vi "Two Color Calibration.vi"(7 "Calling VI Ref":refnum<vi>) -> ()   [LabVIEW 2016]
uses:
  <vilib>/Utility/miscctls.llb/LVPointTypeDef.ctl
  Hardware Configuration/Hardware Configuration Controls/Device Type.ctl
  Hardware Configuration/Hardware Configuration Controls/Device Function.ctl
  Two Color Cal Type Defs/Two Color Cal Notifier Type.ctl
  Two Color Cal Type Defs/Two Color Cal Actions.ctl
  Tools/TIFF Image Read and Write/ImageJ TIF Type Defs/TIF Write Image Information.ctl
  Device Library/Cameras/Camera Controls/Generic Camera Actions.ctl
  Device Library/AOTFs/AOTF Controls/AOTF Actions.ctl
  Device Library/Stages/Stages Controls/Stage Actions.ctl
  shell32.dll
panel:
  in  "Number of Y Steps":u16=10
  out "Current Y Step":u16
  out "Current X Step":u16
  in  "Number of X Steps":u16=10
  in  "Step Size (µm)":dbl=2.0
  in  "Start":bool
  in  "Quit":bool
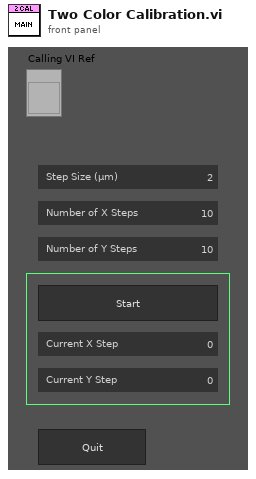
[diagram p1: front panel]
types:
  T1 = typedef "Device Function.ctl" = enum16{"Primary", "Secondary", "Overview", "Wide Field Drift Correction", "642 nm Excitation", "560 nm Excitation", "940 nm Excitation", "546 nm Excitation", "488 nm Excitation", "405 nm Excitation", "Objective Drift Correction", "4Pi Objective Lock", "Objective XY", "Objective Z", "Sample XY", "Sample Coarse Z", "Sample Z", "4Pi Lower", "4Pi Upper", "Mojo", "Adj Cavity", "Line Scanning", "Alert"}
  T2 = typedef "Device Type.ctl" = enum16{"AOTF", "Camera", "Deformable Mirror", "Laser", "Shutter", "Stage", "Waveform", "FPGA", "Email"}
  T3 = typedef "Two Color Cal Actions.ctl" = enum16{"Idle", "Start", "Open FIle", "Laser On", "Start Camera", "Capture", "Move XY", "Abort", "Quit"}
  T4 = typedef "Two Color Cal Notifier Type.ctl" = cluster{"Actions":T3, "X Steps":u16, "Y Steps":u16, "Save File Path":path, "Save File Ref":refnum<file>}
  T5 = enum16{"Always On", "Always Off", "Off While Running"}
  T6 = typedef "LVPointTypeDef.ctl" = cluster{"Horizontal":i16, "Vertical":i16}
  T7 = typedef "Generic Camera Actions.ctl" = enum16{"Status", "Live Preview", "Capture", "Abort", "Set Exposure Time (s)", "Get Exposure Time (s)", "Record Settings", "Set ROI", "Get ROI", "Defect Correction On/Off", "Cooler On/Off", "Fan On/Off", "Quti"}
  T8 = typedef "TIF Write Image Information.ctl" = cluster{"Image Width (Pixels)":u32, "Image Height (Pixels)":u32, "Pixel Width (µm)":dbl, "Pixel Height (µm)":dbl, "Bits Per Sample (e.g. 16)":u32, "No. of Frames":u32, "No. of Slices":u32, "Time Step (sec)":dbl, "Z Step (µm)":dbl}
  T9 = typedef "AOTF Actions.ctl" = enum16{"Error Check", "Blank", "Line On/Off", "Set Power", "Status", "Quit"}
  T10 = typedef "Stage Actions.ctl" = enum16{"Get Position", "MVR", "MOVE", "HALT", "ONTARGET", "ERROR", "REFERENCE", "INIT", "VELOCITY", "STATUS", "EXIT", "HOME", "ZEROPOS", "NANOPOS", "ANALOG", "QUIT"}
  T11 = enum32{"Invalid", "Standard", "Closed", "Hidden", "Minimized", "Maximized"}
  T12 = typedef "IMAQ Image.ctl" = refnum<image>
  T13 = typedef "Camera IMAQ Key Info.ctl" = cluster{"Frame":u32, "Sensor Height":i32, "Sensor Width":i32, "ROI Height":i32, "ROI Width":i32, "ROI Enable?":bool, "Bit per Pixel":u8}
  T14 = typedef "LVRectTypeDef.ctl" = cluster{"Left":i16, "Top":i16, "Right":i16, "Bottom":i16}
  T15 = typedef "LVBoundsTypeDef.ctl" = cluster{"Width":u32, "Height":u32}
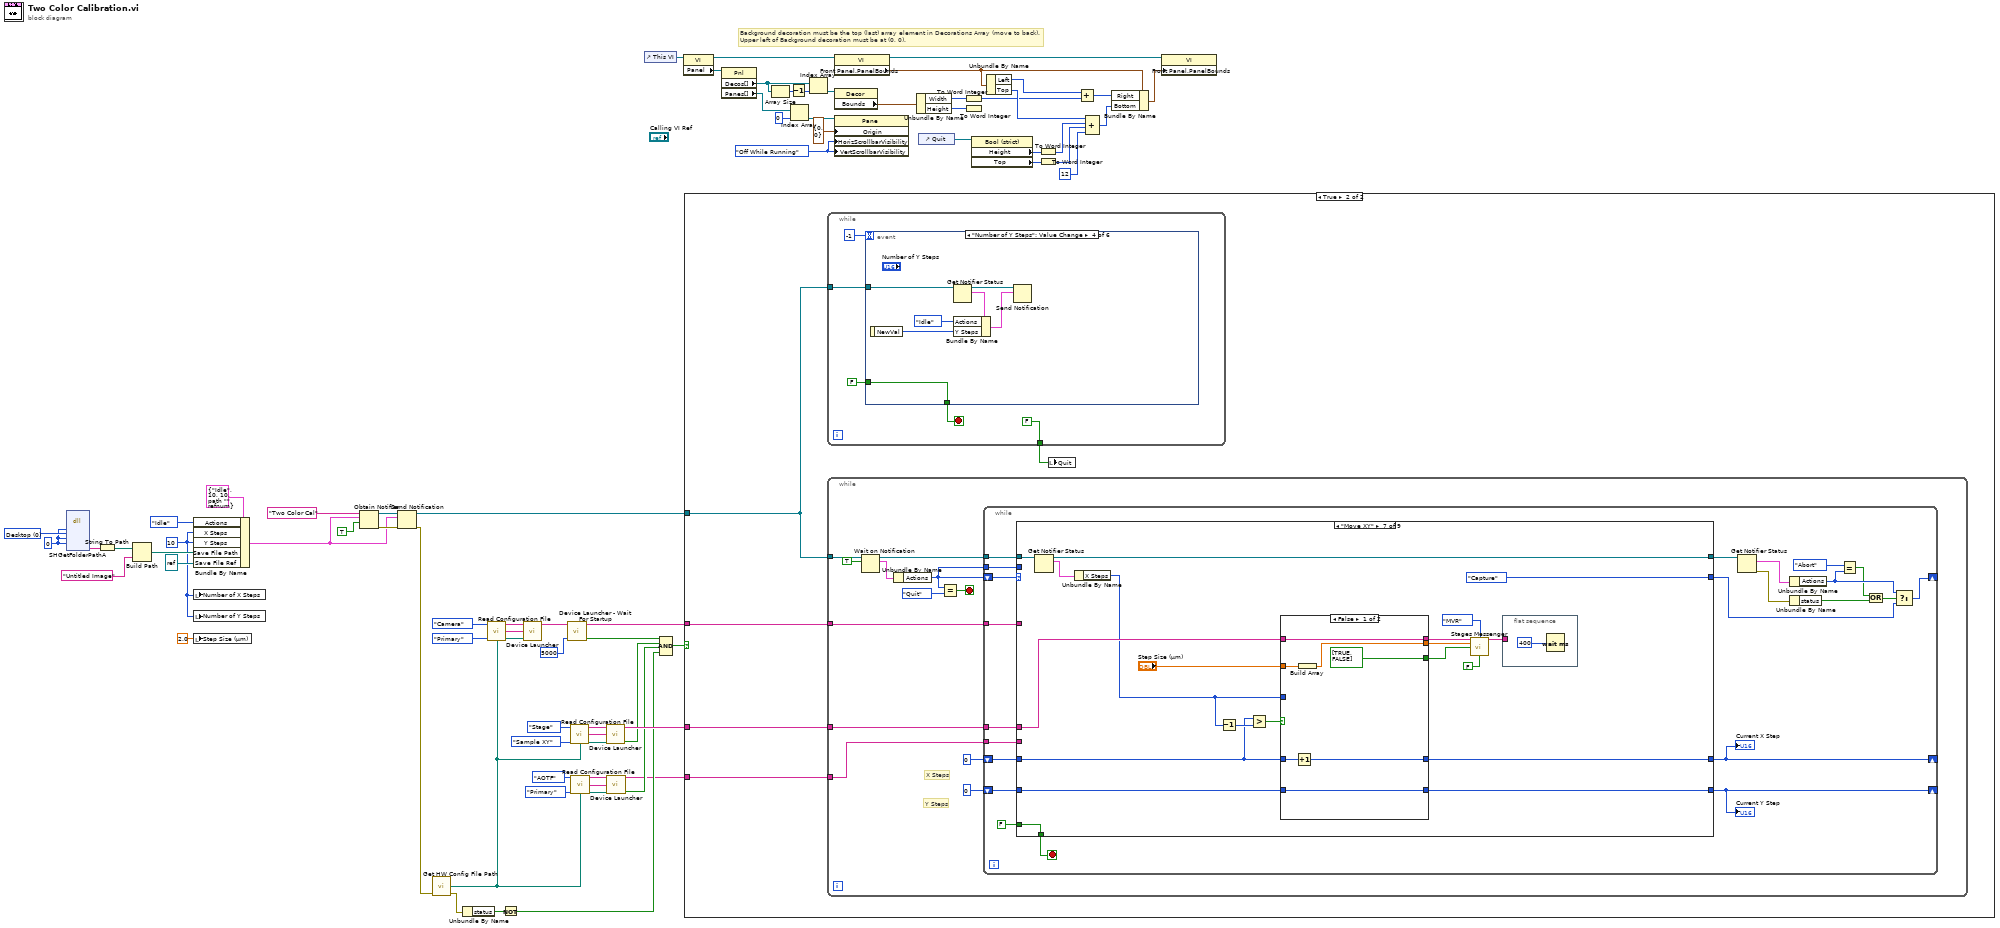
[diagram p0: block diagram]
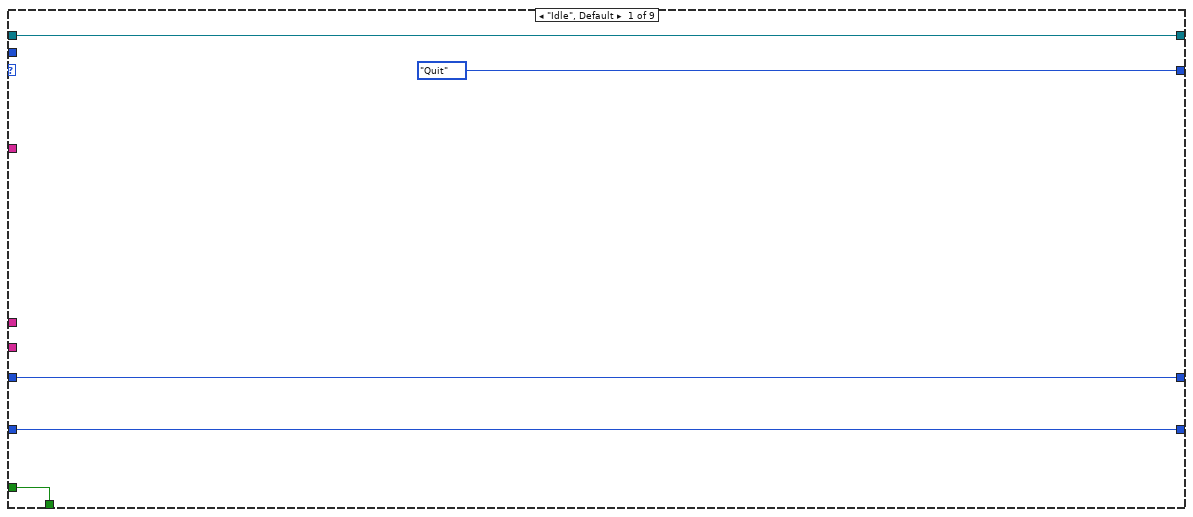
[diagram p3: hidden frame]
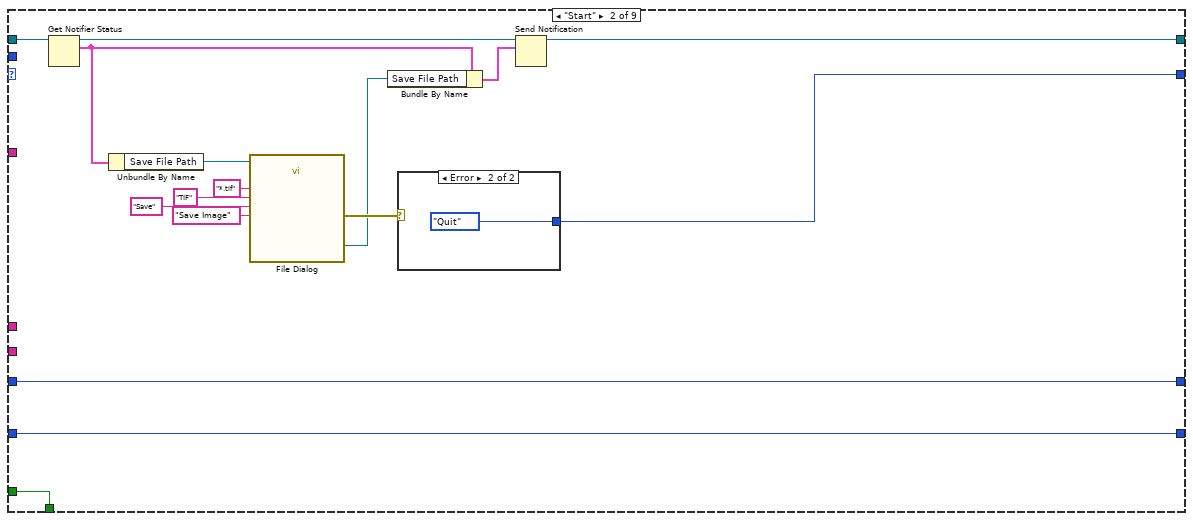
[diagram p4: hidden frame]
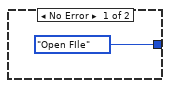
[diagram p5: hidden frame]
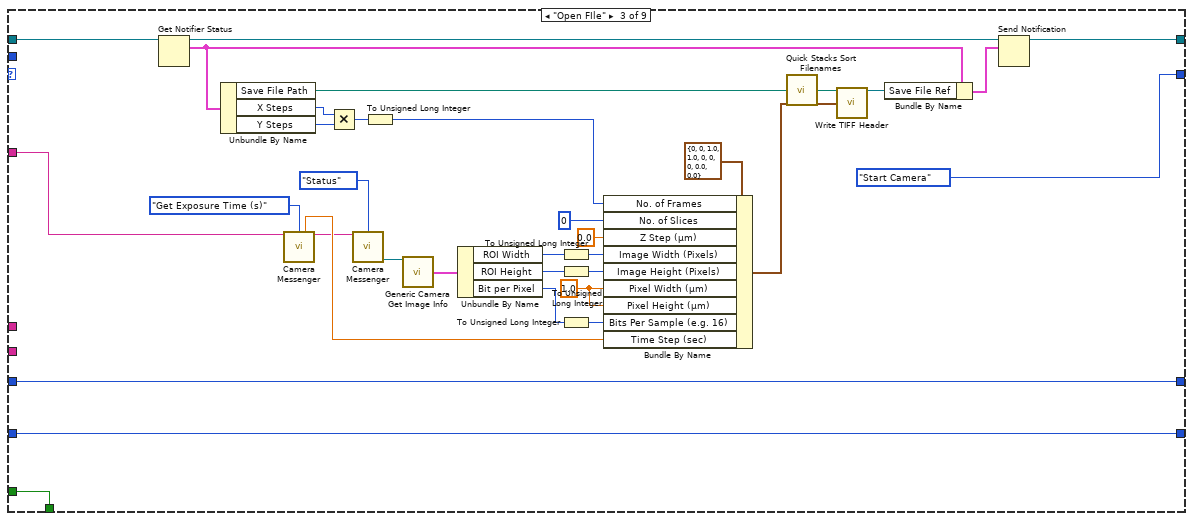
[diagram p6: hidden frame]
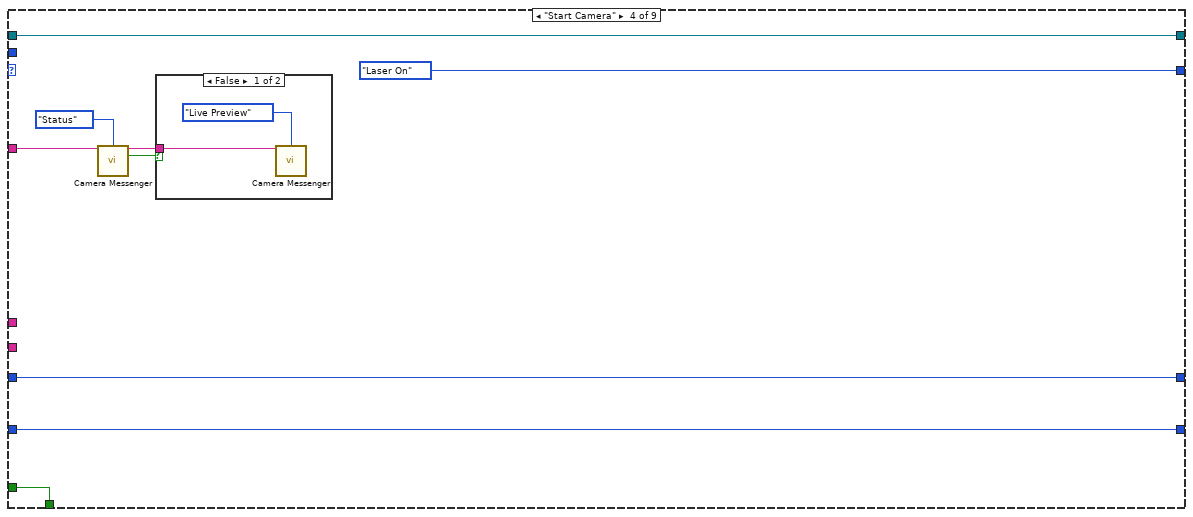
[diagram p7: hidden frame]
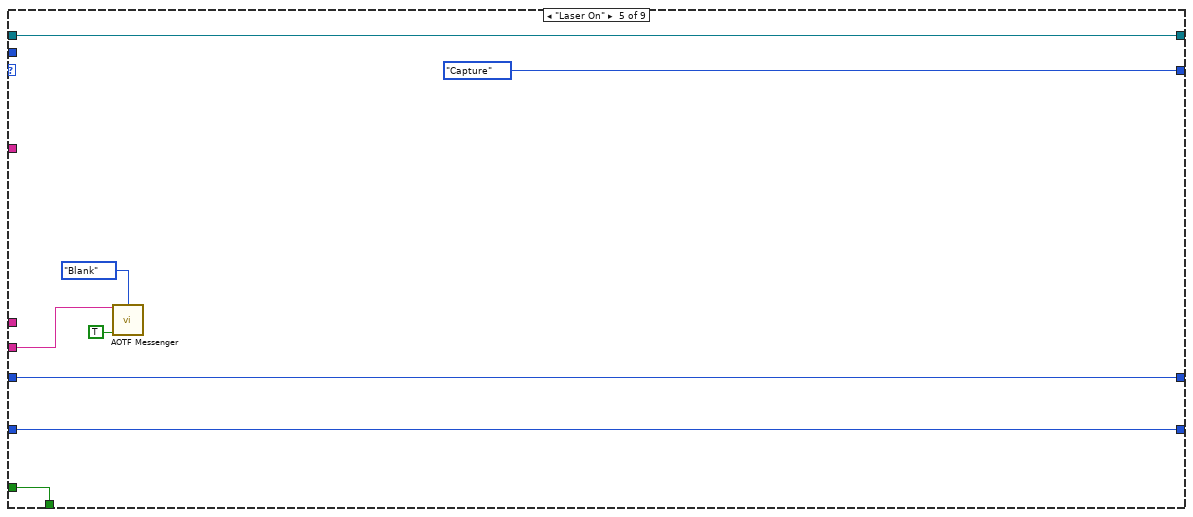
[diagram p9: hidden frame]
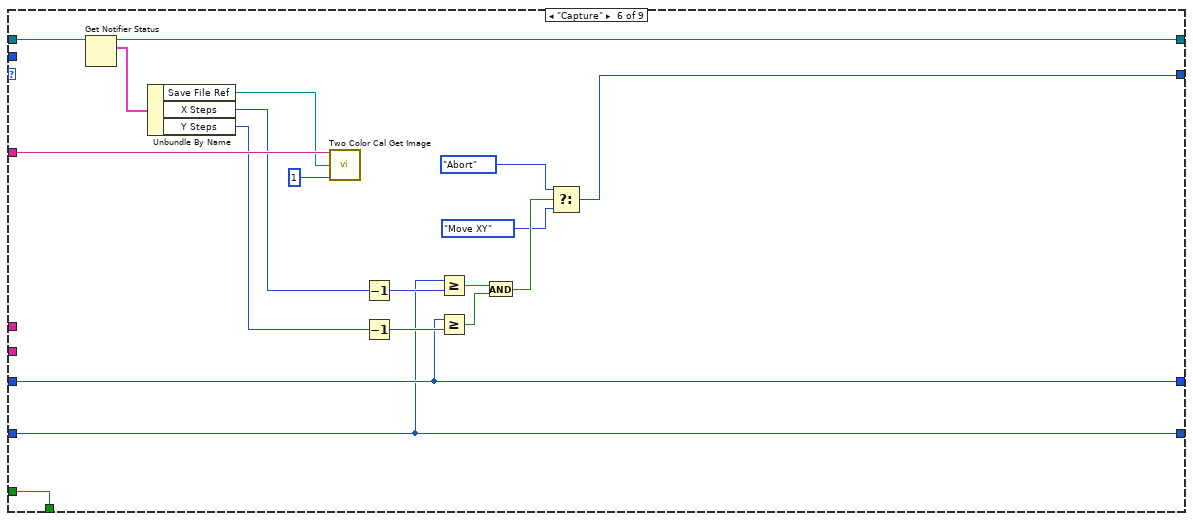
[diagram p10: hidden frame]
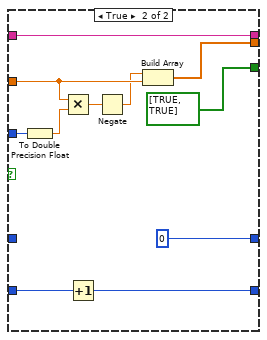
[diagram p11: hidden frame]
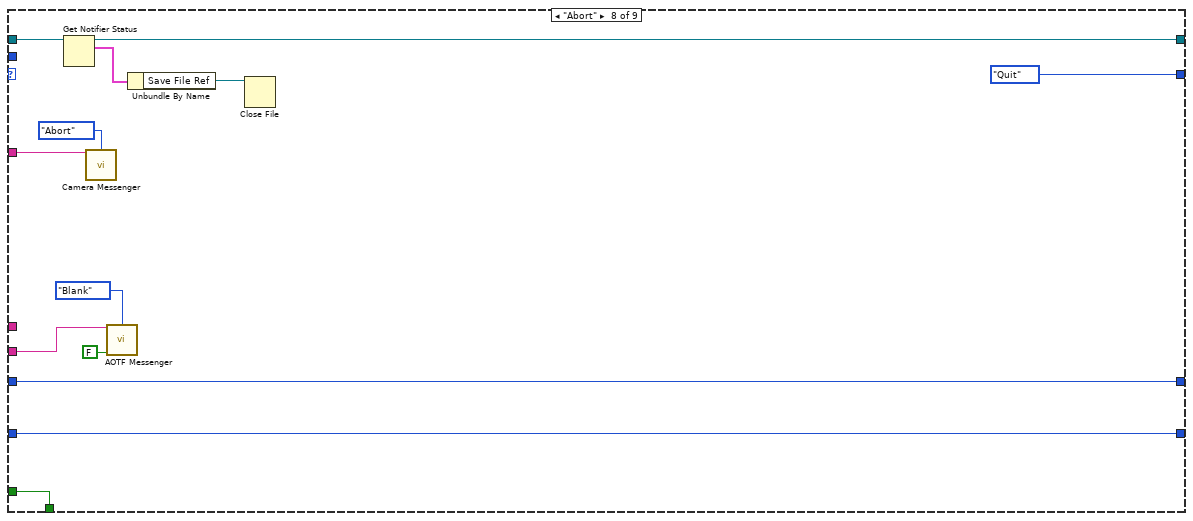
[diagram p12: hidden frame]
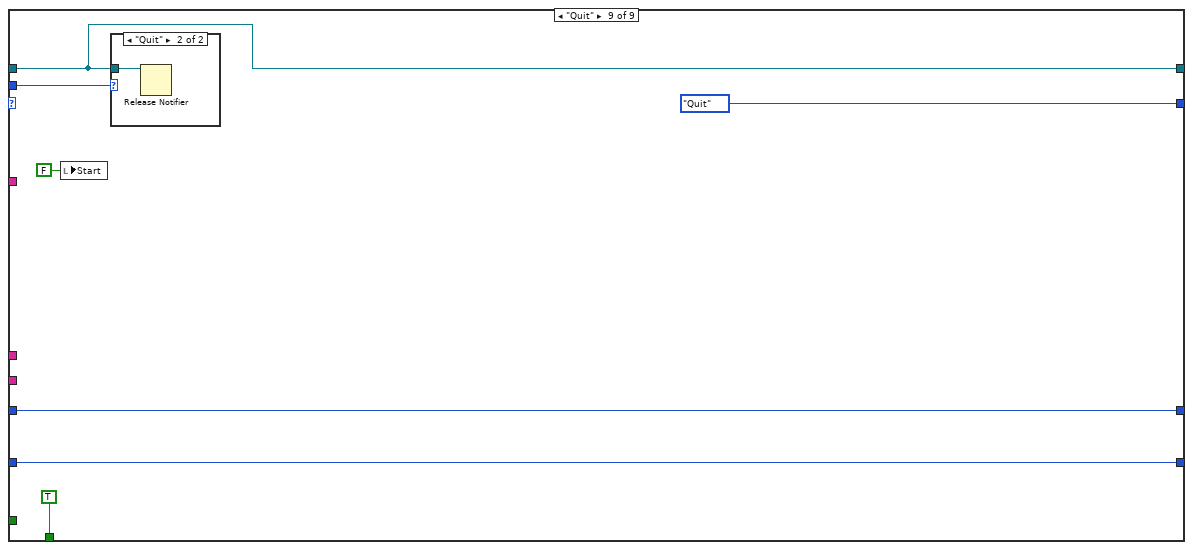
[diagram p13: hidden frame]
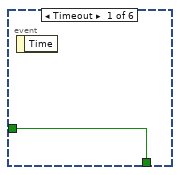
[diagram p15: hidden frame]
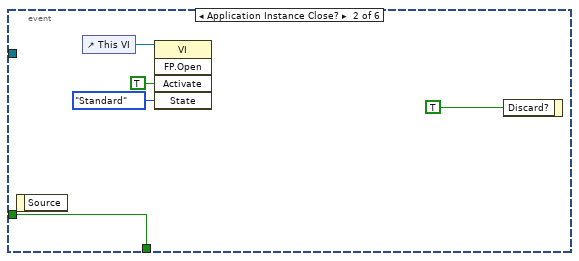
[diagram p16: hidden frame]
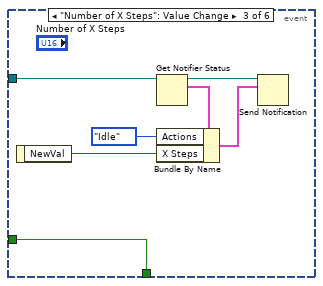
[diagram p17: hidden frame]
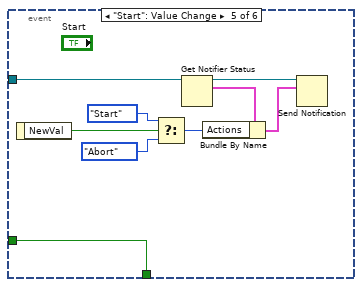
[diagram p18: hidden frame]
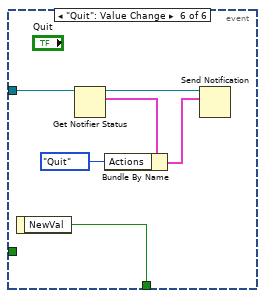
[diagram p19: hidden frame]
diagram:
  w2 = u16 10 ("Y Steps")
  w21 = 0 items=["Desktop"=0, "Personal Documents"=5, "AppData"=26, "Local AppData"=28, "Common AppData"=35, "Program Files"=38, "Program Files Common"=43, "Common Documents"=46] ("Requested Path")
  w20 = 0 ("HWND")
  w58 = T5."Off While Running" ("Vertical Scrollbar Visibility")
  # "Background decoration must be the top (last) array element in Decorations Array (move to back).\nUpper left of Background decoration must be at (0, 0)."
  n1 = dll-call lib="shell32.dll" fn="SHGetFolderPathA"("HWND"=w20, "nFolder"=w21, "hToken"=w20, "dwFlags"=w20) -> ("pszPath"=w19:string)  [unwired: 9 in, 2 out]
  n2 = String To Path(string=w19) -> (path=w17:path)
  n3 = Build Path(base path=w17, name or relative path="Untitled Image") -> (appended path=w14:path)
  n4 = Bundle By Name(cluster=T4 {"Actions"=enum."Idle", "X Steps"=10, "Y Steps"=10, "Save File Path"=path "", "Save File Ref"=refnum} ("Two Color Notifier Type"), "Actions"=Two_Color_Cal_Actions."Idle", "X Steps"=w2, "Y Steps"=w2, "Save File Path"=w14, "Save File Ref"=refnum<file> refnum) -> (w12:T4)
  n5 = local write "Number of X Steps"(w2) -> ()
  n6 = local write "Number of Y Steps"(w2) -> ()
  n7 = local write "Step Size (µm)"(2.0 ("Step Size (µm)")) -> ()
  n8 = Obtain Notifier(name (unnamed)="Two Color Cal", notification data type=w12, create if not found? (T)=TRUE) -> (notifier out=w44:refnum<notifier>, error out=w43:errorcluster)  [unwired: 1 in, 1 out]
  n9 = Send Notification(notification=w12, notifier=w44, error in (no error)=w43) -> (notifier out=w42:refnum<notifier>, error out=w41:errorcluster)
  n10 = call "Get HW Config File Path.vi"("Error"=w41) -> ("File Path"=w6:path, "Error"=w27:errorcluster)  [unwired: 13 in]
  n11 = Unbundle By Name(w27) -> ("status"=w26:bool)
  n12 = call "Read Configuration File.vi"("Device Type"=Device_Type."Camera", "Device Function"=Device_Function."Primary", "Config File Path"=w6) -> ("Unique Notifier Name"=w38:string, "Device Ports/IDs/Channels"=w40:string[], "Device Engine Path"=w39:path)  [unwired: 9 in, 1 out]
  n13 = Not(x=w26) -> (.not. x?=w4:bool)
  n14 = call "Device Launcher.vi"("Notifier Name"=w38, "Device Ports/IDs/Channels"=w40, "Device Engine Path"=w39) -> ("Notifier Name"=w36:string)  [unwired: 11 in, 1 out]
  n15 = call "Device Launcher - Wait For Startup.vi"("Notifier Name"=w36, "Wait Time (ms)"=5000) -> ("Notifier Name (Dup)"=w22:string, "Running?"=w25:bool)  [unwired: 12 in]
  n16 = call "Read Configuration File.vi"("Device Type"=Device_Type."Stage", "Device Function"=Device_Function."Sample XY", "Config File Path"=w6) -> ("Unique Notifier Name"=w31:string, "Device Ports/IDs/Channels"=w29:string[], "Device Engine Path"=w30:path)  [unwired: 9 in, 1 out]
  n17 = call "Read Configuration File.vi"("Device Type"=Device_Type."AOTF", "Device Function"=Device_Function."Primary", "Config File Path"=w6) -> ("Unique Notifier Name"=w11:string, "Device Ports/IDs/Channels"=w9:string[], "Device Engine Path"=w10:path)  [unwired: 9 in, 1 out]
  n18 = call "Device Launcher.vi"("Notifier Name"=w31, "Device Ports/IDs/Channels"=w29, "Device Engine Path"=w30) -> ("Notifier Name"=w28:string, "Running?"=w24:bool)  [unwired: 11 in]
  n19 = call "Device Launcher.vi"("Notifier Name"=w11, "Device Ports/IDs/Channels"=w9, "Device Engine Path"=w10) -> ("Notifier Name"=w3:string, "Running?"=w5:bool)  [unwired: 11 in]
  n20 = control-ref of="This VI"() -> (w50:refnum<vi>)
  n21 = Compound Arithmetic op=AND(w25, w24, w5, w4) -> (w23:bool)
  n22 = property class="VI"(reference=w50) -> (reference out=w59:refnum<vi>, "Panel"=w51:refnum<vi>)  [unwired: 1 in, 1 out]
  n23 = case shown="True" w23 {
    tunnel: w42 -> [_ w79]
    tunnel: w28 -> [_ w78]
    tunnel: w22 -> [_ w77]
    tunnel: w3 -> [_ w76]
    frame False {
    }
    frame True {
      n24 = while {
        tunnel: [FALSE] -> w80
        tunnel: w79 -> [w270]
        stop <- w272 stop-if-true
        n25 = event shown="[3] \"Number of Y Steps\": Value Change" {
          selector: _ -> [_ _ _ _ _ _]
          dyn-events: _ -> [_ _ _ _ _ _]
          timeout: -1 -> [_ _ _ _ _ _]
          tunnel: FALSE -> [w275 w279 w287 w294 w303 _]
          tunnel: [w275 w279 w287 w294 w303 w309] -> w272
          tunnel: w270 -> [_ _ w286 w293 w301 w307]
          event Timeout {
            n26 = event-data() -> ()  [unwired: 1 in, 1 out]
          }
          event Application Instance Close? {
            n27 = event-data() -> ()  [unwired: 1 in, 1 out]
            n28 = control-ref of="This VI"() -> (w276:refnum<vi>)
            n29 = invoke class="VI" method="FP.Open"(reference=w276, "Activate"=TRUE ("Activate?"), "State"=T11."Standard") -> ()  [unwired: 2 in, 5 out]
            n30 = event-data("Discard?"=TRUE) -> ()  [unwired: 1 in, 1 out]
          }
          event "Number of X Steps": Value Change {
            n31 = event-data() -> ("NewVal"=w281:u16)  [unwired: 1 in]
            n32 = Get Notifier Status(notifier=w286) -> (notifier out=w283:refnum<notifier>, current notification=w285:T4)  [unwired: 1 in, 3 out]
            n33 = Bundle By Name(cluster=w285, "Actions"=Two_Color_Cal_Actions."Idle", "X Steps"=w281) -> (w282:T4)
            n34 = Send Notification(notification=w282, notifier=w283) -> ()  [unwired: 1 in, 2 out]
          }
          event "Number of Y Steps": Value Change {
            n35 = event-data() -> ("NewVal"=w288:u16)  [unwired: 1 in]
            n36 = Get Notifier Status(notifier=w293) -> (notifier out=w290:refnum<notifier>, current notification=w292:T4)  [unwired: 1 in, 3 out]
            n37 = Bundle By Name(cluster=w292, "Actions"=Two_Color_Cal_Actions."Idle", "Y Steps"=w288) -> (w289:T4)
            n38 = Send Notification(notification=w289, notifier=w290) -> ()  [unwired: 1 in, 2 out]
          }
          event "Start": Value Change {
            n39 = event-data() -> ("NewVal"=w298:bool)  [unwired: 1 in]
            n40 = Select(t=Two_Color_Cal_Actions."Start" ("Actions"), s=w298, f=Two_Color_Cal_Actions."Abort" ("Actions")) -> (s? t:f=w295:T3)
            n41 = Get Notifier Status(notifier=w301) -> (notifier out=w302:refnum<notifier>, current notification=w300:T4)  [unwired: 1 in, 3 out]
            n42 = Bundle By Name(cluster=w300, "Actions"=w295) -> (w299:T4)
            n43 = Send Notification(notification=w299, notifier=w302) -> ()  [unwired: 1 in, 2 out]
          }
          event "Quit": Value Change {
            n44 = event-data() -> ("NewVal"=w309:bool)  [unwired: 1 in]
            n45 = Get Notifier Status(notifier=w307) -> (notifier out=w308:refnum<notifier>, current notification=w306:T4)  [unwired: 1 in, 3 out]
            n46 = Bundle By Name(cluster=w306, "Actions"=Two_Color_Cal_Actions."Quit") -> (w304:T4)
            n47 = Send Notification(notification=w304, notifier=w308) -> ()  [unwired: 1 in, 2 out]
          }
        }
      }
      n48 = while {
        tunnel: w78 -> [w87]
        tunnel: w79 -> [w92]
        tunnel: w77 -> [w84]
        tunnel: w76 -> [w81]
        stop <- w89 stop-if-true
        # "Y Steps"
        # "X Steps"
        n49 = Wait on Notification(notifier=w92, ignore previous (F)=TRUE) -> (notifier out=w88:refnum<notifier>, notification=w83:T4)  [unwired: 2 in, 2 out]
        n50 = Unbundle By Name(w83) -> ("Actions"=w82:T3)
        n51 = Equal?(x=w82, y=Two_Color_Cal_Actions."Quit") -> (x = y?=w89:bool)
        n52 = while {
          tunnel: w88 -> [w114]
          tunnel: w87 -> [w110]
          tunnel: w82 -> [w109]
          shift-right: [w93] -> _
          shift-left: w82 -> [w113]
          shift-right: [w106] -> _
          shift-left: u16 0 -> [w108]
          shift-right: [w105] -> _
          shift-left: u16 0 -> [w107]
          tunnel: w84 -> [w104]
          tunnel: w81 -> [w103]
          stop <- w111 stop-if-true
          n53 = case shown="\"Move XY\"" w113 {
            tunnel: w114 -> [w115 w132 w168 w174 w187 w197 w212 w258 w262]
            tunnel: FALSE -> [w119 w135 w171 w180 w189 w209 w228 w261 _]
            tunnel: [w119 w135 w171 w180 w189 w209 w228 w261 TRUE] -> w111
            tunnel: w110 -> [_ _ _ _ _ _ w225 _ _]
            tunnel: w109 -> [_ _ _ _ _ _ _ _ w267]
            tunnel: [Two_Color_Cal_Actions."Quit" ("y") w121 Two_Color_Cal_Actions."Start Camera" ("y") Two_Color_Cal_Actions."Laser On" ("y") Two_Color_Cal_Actions."Capture" ("y") w207 Two_Color_Cal_Actions."Capture" ("y") Two_Color_Cal_Actions."Quit" ("y") Two_Color_Cal_Actions."Quit" ("y")] -> w94
            tunnel: w108 -> [w117 w134 w170 w179 w184 w201 w223 w260 w265]
            tunnel: w107 -> [w116 w133 w169 w178 w183 w200 w216 w259 w264]
            tunnel: [w117 w134 w170 w179 w184 w201 w222 w260 w265] -> w106
            tunnel: [w116 w133 w169 w178 w183 w200 w215 w259 w264] -> w105
            tunnel: w104 -> [_ _ w138 w175 _ w199 _ w250 _]
            tunnel: [w115 w120 w166 w174 w187 w192 w210 w257 w262] -> w95
            tunnel: w103 -> [_ _ _ _ w188 _ _ w252 _]
            frame "Idle", Default {
            }
            frame "Start" {
              n54 = Get Notifier Status(notifier=w132) -> (notifier out=w131:refnum<notifier>, current notification=w130:T4)  [unwired: 1 in, 3 out]
              n55 = Unbundle By Name(w130) -> ("Save File Path"=w128:path)
              n56 = call "File Dialog"("start path"=w128, "prompt"="Save Image", "button label"="Save", "pattern (all files)"="*.tif", "pattern label"="TIF") -> ("selected path"=w122:path, "error out"=w127:errorcluster)  [unwired: 7 in, 2 out]
              n57 = Bundle By Name(cluster=w130, "Save File Path"=w122) -> (w129:T4)
              n58 = case shown="Error" w127 {
                tunnel: [Two_Color_Cal_Actions."Open FIle" ("y") Two_Color_Cal_Actions."Quit" ("y")] -> w121
                frame No Error {
                }
                frame Error {
                }
              }
              n59 = Send Notification(notification=w129, notifier=w131) -> (notifier out=w120:refnum<notifier>)  [unwired: 1 in, 1 out]
            }
            frame "Open FIle" {
              w159 = 1.0 ("Pixel Width (µm)")
              n60 = Get Notifier Status(notifier=w168) -> (notifier out=w140:refnum<notifier>, current notification=w142:T4)  [unwired: 1 in, 3 out]
              n61 = Unbundle By Name(w142) -> ("Save File Path"=w146:path, "X Steps"=w150:u16, "Y Steps"=w149:u16)
              n62 = call "Camera Messenger.vi"("Notifier Name"=w138, "General Camera Actions"=Generic_Camera_Actions."Get Exposure Time (s)") -> ("Current Exposure Time (s)"=w163:dbl, "Notifier Name Dup"=w162:string)  [unwired: 8 in, 4 out]
              n63 = Multiply(x=w150, y=w149) -> (x*y=w148:u16)
              n64 = call "Camera Messenger.vi"("Notifier Name"=w162, "General Camera Actions"=Generic_Camera_Actions."Status") -> ("Image Ref"=w154:T12)  [unwired: 8 in, 5 out]
              n65 = To Unsigned Long Integer(number=w148) -> (unsigned 32bit integer=w147:u32)
              n66 = call "Generic Camera Get Image Info.vi"("Image Ref"=w154) -> ("Camera Image Info"=w155:T13)  [unwired: 14 in]
              n67 = Unbundle By Name(w155) -> ("ROI Width"=w156:i32, "ROI Height"=w157:i32, "Bit per Pixel"=w158:u8)
              n68 = To Unsigned Long Integer(number=w156) -> (unsigned 32bit integer=w144:u32)
              n69 = To Unsigned Long Integer(number=w157) -> (unsigned 32bit integer=w143:u32)
              n70 = To Unsigned Long Integer(number=w158) -> (unsigned 32bit integer=w145:u32)
              n71 = Bundle By Name(cluster=T8 {"Image Width (Pixels)"=0, "Image Height (Pixels)"=0, "Pixel Width (µm)"=1.0, "Pixel Height (µm)"=1.0, "Bits Per Sample (e.g. 16)"=0, "No. of Frames"=0, "No. of Slices"=0, "Time Step (sec)"=0.0, "Z Step (µm)"=0.0} ("Image Info"), "No. of Frames"=w147, "No. of Slices"=u32 0, "Z Step (µm)"=0.0, "Image Width (Pixels)"=w144, "Image Height (Pixels)"=w143, "Pixel Width (µm)"=w159, "Pixel Height (µm)"=w159, "Bits Per Sample (e.g. 16)"=w145, "Time Step (sec)"=w163) -> (w153:T8)
              n72 = call "Quick Stacks Sort Filenames.vi"("Requested File Path"=w146) -> ("Resulting File Path"=w151:path)  [unwired: 14 in]
              n73 = call "Write TIFF Header.vi"("File Path"=w151, "Image Info"=w153) -> ("File Ref"=w141:refnum<file>)  [unwired: 11 in, 2 out]
              n74 = Bundle By Name(cluster=w142, "Save File Ref"=w141) -> (w139:T4)
              n75 = Send Notification(notification=w139, notifier=w140) -> (notifier out=w166:refnum<notifier>)  [unwired: 1 in, 1 out]
            }
            frame "Start Camera" {
              n76 = call "Camera Messenger.vi"("Notifier Name"=w175, "General Camera Actions"=Generic_Camera_Actions."Status") -> ("Notifier Name Dup"=w176:string, "Running?"=w172:bool)  [unwired: 8 in, 4 out]
              n77 = case shown="False" w172 {
                tunnel: w176 -> [w182 _]
                frame False {
                  n78 = call "Camera Messenger.vi"("Notifier Name"=w182, "General Camera Actions"=Generic_Camera_Actions."Live Preview") -> ()  [unwired: 8 in, 6 out]
                }
                frame True {
                }
              }
            }
            frame "Laser On" {
              n79 = call "AOTF Messenger.vi"("AOTF Notifier Name"=w188, "AOTF Action"=AOTF_Actions."Blank", "Beam Blank"=TRUE) -> ()  [unwired: 7 in, 6 out]
            }
            frame "Capture" {
              n80 = Get Notifier Status(notifier=w197) -> (notifier out=w192:refnum<notifier>, current notification=w196:T4)  [unwired: 1 in, 3 out]
              n81 = Unbundle By Name(w196) -> ("Save File Ref"=w195:refnum<file>, "X Steps"=w194:u16, "Y Steps"=w193:u16)
              n82 = call "Two Color Cal Get Image.vi"("Notifier Name"=w199, "Write File Ref"=w195, "Num of Frames"=u16 1) -> ()  [unwired: 13 in]
              n83 = Decrement(x=w194) -> (x-1=w206:u16)
              n84 = Decrement(x=w193) -> (x-1=w205:u16)
              n85 = Greater Or Equal?(x=w200, y=w206) -> (x >= y?=w204:bool)
              n86 = Greater Or Equal?(x=w201, y=w205) -> (x >= y?=w203:bool)
              n87 = And(x=w204, y=w203) -> (x .and. y?=w202:bool)
              n88 = Select(t=Two_Color_Cal_Actions."Abort" ("y"), s=w202, f=Two_Color_Cal_Actions."Move XY" ("y")) -> (s? t:f=w207:T3)
            }
            frame "Move XY" {
              n89 = Get Notifier Status(notifier=w212) -> (notifier out=w210:refnum<notifier>, current notification=w213:T4)  [unwired: 1 in, 3 out]
              n90 = Unbundle By Name(w213) -> ("X Steps"=w211:u16)
              n91 = Decrement(x=w211) -> (x-1=w227:u16)
              n92 = Greater?(x=w223, y=w227) -> (0:w226:bool)
              n93 = case shown="False" w226 {
                tunnel: w225 -> [w235 w244]
                tunnel: "Step Size (µm)" -> [w237 w241]
                tunnel: [w236 u16 0] -> w222
                tunnel: w223 -> [w232 _]
                tunnel: [w235 w244] -> w219
                tunnel: [w234 w245] -> w218
                tunnel: [bool[] [TRUE, FALSE] ("Axis") bool[] [TRUE, TRUE] ("Axis")] -> w217
                tunnel: w211 -> [_ w242]
                tunnel: w216 -> [w231 w239]
                tunnel: [w231 w238] -> w215
                frame False {
                  n94 = Increment(x=w232) -> (x+1=w236:u16)
                  n95 = Build Array(w237) -> (w234:dbl[])
                }
                frame True {
                  n96 = To Double Precision Float(number=w242) -> (double precision float=w247:dbl)
                  n97 = Multiply(x=w241, y=w247) -> (x*y=w246:dbl)
                  n98 = Increment(x=w239) -> (x+1=w238:u16)
                  n99 = Negate(x=w246) -> (-x=w240:dbl)
                  n100 = Build Array(w240, w241) -> (w245:dbl[])
                }
              }
              n101 = call "Stages Messenger.vi"("Stage Notifier Name"=w219, "Actions"=Stage_Actions."MVR", "Setpoint"=w218, "Axis"=w217, "Exit While Busy?"=FALSE) -> ("Stage Notifier Name (Dup)"=w214:string)  [unwired: 7 in, 3 out]
              n102 = flat-sequence {
                tunnel: w214 -> [_]
                frame #0 {
                  n103 = Wait (ms)(milliseconds to wait=u32 400 ("Stage Delay")) -> ()  [unwired: 1 out]
                }
              }
            }
            frame "Abort" {
              n104 = Get Notifier Status(notifier=w258) -> (notifier out=w257:refnum<notifier>, current notification=w256:T4)  [unwired: 1 in, 3 out]
              n105 = call "Camera Messenger.vi"("Notifier Name"=w250, "General Camera Actions"=Generic_Camera_Actions."Abort") -> ()  [unwired: 8 in, 6 out]
              n106 = call "AOTF Messenger.vi"("AOTF Notifier Name"=w252, "AOTF Action"=AOTF_Actions."Blank", "Beam Blank"=FALSE) -> ()  [unwired: 7 in, 6 out]
              n107 = Unbundle By Name(w256) -> ("Save File Ref"=w255:refnum<file>)
              n108 = Close File(refnum=w255) -> ()  [unwired: 1 in, 2 out]
            }
            frame "Quit" {
              n109 = local write "Start"(FALSE ("Start")) -> ()
              n110 = case shown="\"Quit\"" w267 {
                tunnel: w262 -> [_ w269]
                frame Default {
                }
                frame "Quit" {
                  n111 = Release Notifier(notifier=w269) -> ()  [unwired: 2 in, 3 out]
                }
              }
            }
          }
          "Current Y Step" <- w105
          "Current X Step" <- w106
          n112 = Get Notifier Status(notifier=w95) -> (current notification=w96:T4, error out=w97:errorcluster)  [unwired: 1 in, 3 out]
          n113 = Unbundle By Name(w96) -> ("Actions"=w102:T3)
          n114 = Unbundle By Name(w97) -> ("status"=w99:bool)
          n115 = Equal?(x=Two_Color_Cal_Actions."Abort", y=w102) -> (x = y?=w100:bool)
          n116 = Or(x=w100, y=w99) -> (x .or. y?=w101:bool)
          n117 = Select(t=w102, s=w101, f=w94) -> (s? t:f=w93:T3)
        }
      }
      n118 = local write "Quit"(w80) -> ()
    }
  }
  n119 = property class="Pnl"(reference=w51) -> ("Decos[]"=w49:refnum<vi>[], "Panes[]"=w55:refnum<vi>[])  [unwired: 1 in, 2 out]
  n120 = Array Size(array=w49) -> (size(s)=w47:i32)
  n121 = Decrement(x=w47) -> (x-1=w48:i32)
  n122 = Index Array(array=w55, index=0) -> (element=w54:refnum<vi>)
  n123 = Index Array(array=w49, index=w48) -> (element=w57:refnum<vi>)
  n124 = property class="VI"(reference=w59) -> (reference out=w61:refnum<vi>, "Front Panel.PanelBounds"=w62:T14)  [unwired: 1 in, 1 out]
  n125 = property class="Decor"(reference=w57) -> ("Bounds"=w60:T15)  [unwired: 1 in, 2 out]
  n126 = property class="Pane"(reference=w54, "Origin"=T6 {"Horizontal"=0, "Vertical"=0}, "HorizScrollbarVisibility"=w58, "VertScrollbarVisibility"=w58) -> ()  [unwired: 1 in, 2 out]
  n127 = Unbundle By Name(w60) -> ("Width"=w65:u32, "Height"=w68:u32)
  n128 = control-ref of="Quit"() -> (w52:refnum<vi>)
  n129 = To Word Integer(number=w65) -> (16bit integer=w67:i16)
  n130 = To Word Integer(number=w68) -> ()  [unwired: 1 out]
  n131 = property class="Bool (strict)"(reference=w52) -> ("Height"=w70:u32, "Top"=w71:i32)  [unwired: 1 in, 2 out]
  n132 = Unbundle By Name(w62) -> ("Left"=w64:i16, "Top"=w75:i16)
  n133 = To Word Integer(number=w70) -> (16bit integer=w73:i16)
  n134 = To Word Integer(number=w71) -> (16bit integer=w74:i16)
  n135 = Add(x=w64, y=w67) -> (x+y=w66:i16)
  n136 = Compound Arithmetic op=ADD(w75, w73, w74, i16 12 ("y")) -> (w69:i16)
  n137 = Bundle By Name(cluster=w62, "Right"=w66, "Bottom"=w69) -> (w63:T14)
  n138 = property class="VI"(reference=w61, "Front Panel.PanelBounds"=w63) -> ()  [unwired: 1 in, 2 out]
